vi "Write DAC.vi"(8 "error in (no error)":errorcluster, 10 "Analog Output":u16, 11 "AO in":refnum<class "An Out I2C 1 Chan.lvclass">) -> (0 "error out":errorcluster, 3 "AO out":refnum<class "An Out I2C 1 Chan.lvclass">)   [LabVIEW 2020, in "CTI-Peripheral.lvlib" / "An Out I2C 1 Chan.lvclass"]
uses:
  An Out I2C 1 Chan.lvclass
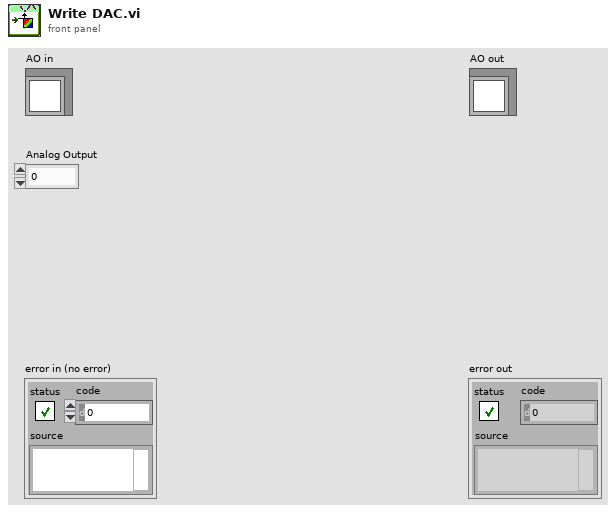
[diagram p1: front panel]
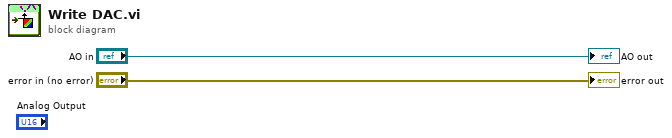
[diagram p0: block diagram]
diagram:
  "error out" <- "error in (no error)"
  "AO out" <- "AO in"
